vi "musik.vi"   [LabVIEW 2016]
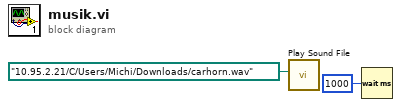
[diagram p0: block diagram]
diagram:
  n1 = call <vilib>:"Play Sound File.vi"("path"=path "10.95.2.21/C/Users/Michi/Downloads/carhorn.wav") -> ()  [unwired: 9 in, 2 out]
  n2 = Wait (ms)(milliseconds to wait=u32 1000) -> ()  [unwired: 1 out]
